vi "getLastChar.vi"(1 "string":string) -> (0 "last char":string)   [LabVIEW 2015]
doc: "returns the last character of <b>string</b>."
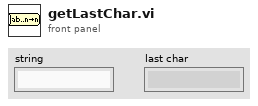
[diagram p1: front panel]
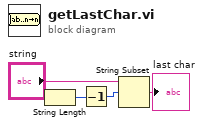
[diagram p0: block diagram]
diagram:
  n1 = String Length(string="string") -> (length=w2:i32)
  n2 = Decrement(x=w2) -> (x-1=w1:i32)
  n3 = String Subset(string="string", offset (0)=w1) -> (substring=→"last char":string)  [unwired: 1 in]
